vi "Assertion Failure Message.vi"() -> ()   [LabVIEW 2017, in "Transparent Assertions.Tests.lvlib" / "Assert Not Count.lvlib"]
uses:
  Assert Not Count.lvlib
  src/Transparent Assertions/Transparent Assertions.lvlib
panel:
  out "error out":errorcluster
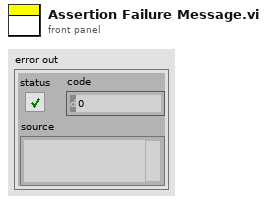
[diagram p1: front panel]
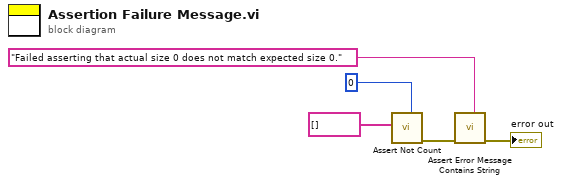
[diagram p0: block diagram]
diagram:
  n1 = call "Assert Not Count.vi"("Expected"=0, "Haystack"=string[] []) -> ("error out"=w5:errorcluster)  [unwired: 9 in]
  n2 = call "Assert Error Message Contains String.vi"("Expected"="Failed asserting that actual size 0 does not match expected size 0." ("y"), "error in (no error)"=w5) -> ("error out"=→"error out":errorcluster)  [unwired: 9 in]
